vi "Stepper eSCL UDP.vi"(8 "error in":errorcluster, 9 "Axis Queue":refnum<queue>, 10 "UI Queue":refnum<queue>) -> (0 "error out":errorcluster)   [LabVIEW 2016, in "SMD-7615.lvlib"]
uses:
  SMD-7615.lvlib
  support/Message Queue/Message Cluster.ctl
  CTL/Stepper Drive Config.ctl
  CTL/SV General.ctl
  CTL/SV Inputs.ctl
  CTL/SV Outputs.ctl
  CTL/Motion IO.ctl
  CTL/Digital Lines (Read).ctl
  CTL/Status.ctl
  CTL/Encoder.ctl
  CTL/Position.ctl
  CTL/Axis Data.ctl
  support/Message Queue/Enqueue Message (Single).vi
  <vilib>/GPower/Error/Library/Append/AppendSingle.vi
  <vilib>/ErrorRing/Error Ring.xnode
  support/Message Queue/Message Queue.lvlib
  <vilib>/GPower/Error/GPError.lvlib
  LUL-All/LUL-Syslog/LUL-SysLog.lvlib
  eSCL/eSCL.lvlib
panel:
  out "DAQ time (ms)":u32
  out "Stall detected (Software)":bool
  out "Moving ? (Software)":bool
  out "Position":T1
  out "Encoder":T2
  out "Status":T3
  in  "Stop Button":bool
  out "Axis Name":string
  out "Digital Lines (Read)":T4
  out "Motion I/O":T5
  out "dt DAQ (ms)":u32
  out "Axis Config Constant":T6
  out "Last Received SV Update":timestamp
  out "Exit ?":bool
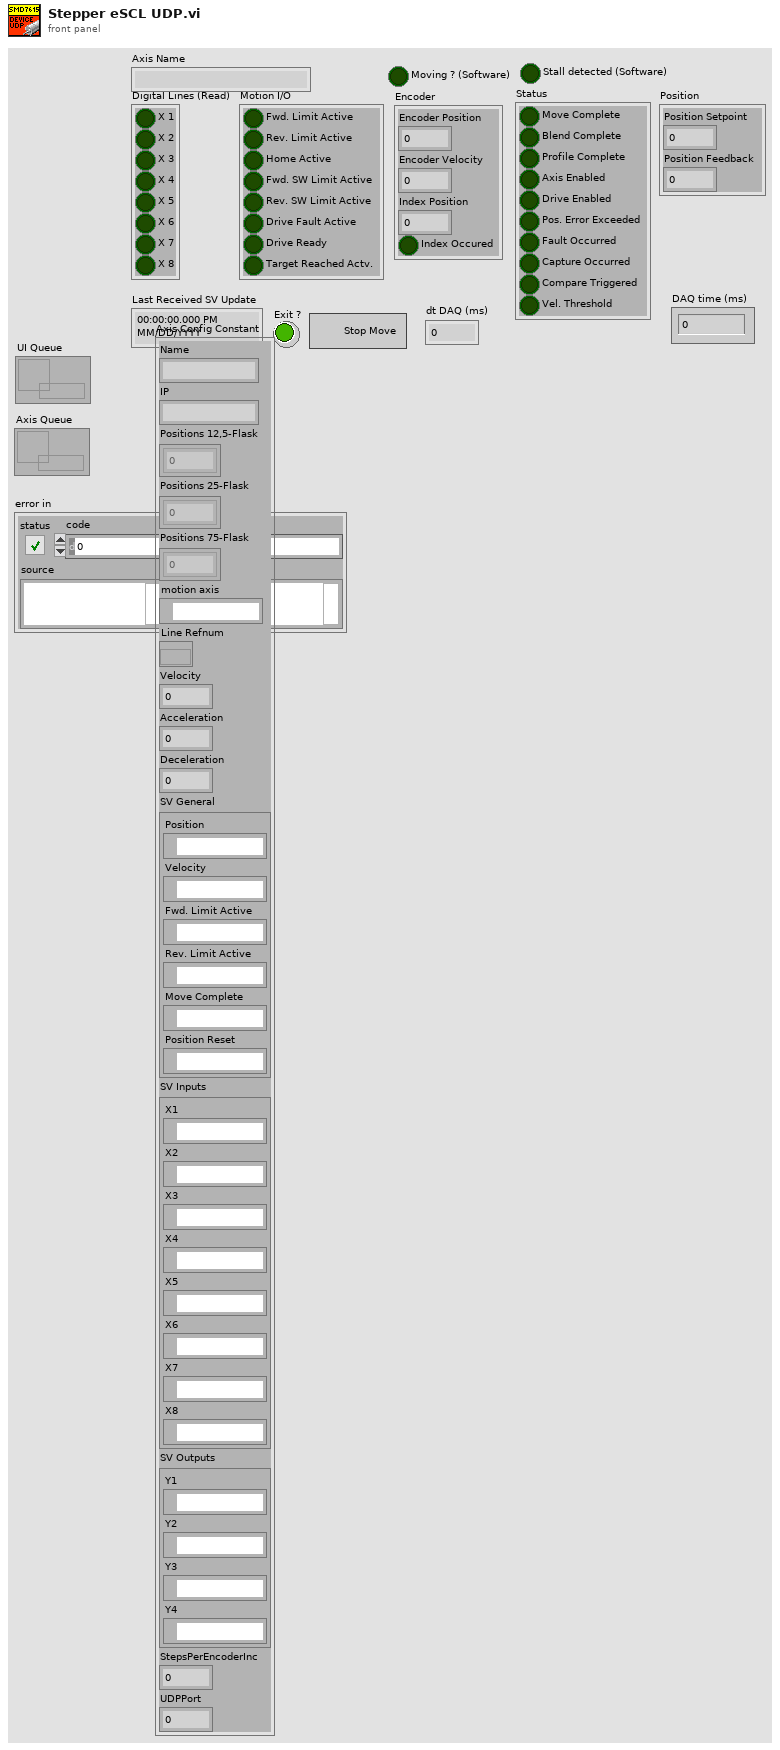
[diagram p1: front panel]
types:
  T1 = typedef "SMD-7615.lvlib/Position.ctl" = cluster{"Position Setpoint":dbl, "Position Feedback":dbl}
  T2 = typedef "SMD-7615.lvlib/Encoder.ctl" = cluster{"Encoder Position":dbl, "Encoder Velocity":dbl, "Index Position":dbl, "Index Occured":bool}
  T3 = typedef "SMD-7615.lvlib/Status.ctl" = cluster{"Move Complete":bool, "Blend Complete":bool, "Profile Complete":bool, "Axis Enabled":bool, "Drive Enabled":bool, "Pos. Error Exceeded":bool, "Fault Occurred":bool, "Capture Occurred":bool, "Compare Triggered":bool, "Vel. Threshold":bool}
  T4 = typedef "SMD-7615.lvlib/Digital Lines (Read).ctl" = cluster{"X 1":bool, "X 2":bool, "X 3":bool, "X 4":bool, "X 5":bool, "X 6":bool, "X 7":bool, "X 8":bool}
  T5 = typedef "SMD-7615.lvlib/Motion IO.ctl" = cluster{"Fwd. Limit Active":bool, "Rev. Limit Active":bool, "Home Active":bool, "Fwd. SW Limit Active":bool, "Rev. SW Limit Active":bool, "Drive Fault Active":bool, "Drive Ready":bool, "Target Reached Actv.":bool}
  T6 = typedef "SMD-7615.lvlib/Stepper Drive Config.ctl" = cluster{"Name":string, "IP":string, "Positions 12,5-Flask":dbl[], "Positions 25-Flask":dbl[], "Positions 75-Flask":dbl[], "motion axis ":refnum<k21>, "Line Refnum":refnum<k20>, "Velocity":dbl, "Acceleration":dbl, "Deceleration":dbl, "SV General":T7, "SV Inputs":T8, "SV Outputs":T9, "StepsPerEncoderInc":i32, "UDPPort":u16}
  T7 = typedef "SMD-7615.lvlib/SV General.ctl" = cluster{"Position":refnum<k21>, "Velocity":refnum<k21>, "Fwd. Limit Active":refnum<k21>, "Rev. Limit Active":refnum<k21>, "Move Complete":refnum<k21>, "Position Reset":refnum<k21>}
  T8 = typedef "SMD-7615.lvlib/SV Inputs.ctl" = cluster{"X1":refnum<k21>, "X2":refnum<k21>, "X3":refnum<k21>, "X4":refnum<k21>, "X5":refnum<k21>, "X6":refnum<k21>, "X7":refnum<k21>, "X8":refnum<k21>}
  T9 = typedef "SMD-7615.lvlib/SV Outputs.ctl" = cluster{"Y1":refnum<k21>, "Y2":refnum<k21>, "Y3":refnum<k21>, "Y4":refnum<k21>}
  T10 = typedef "SMD-7615.lvlib/Axis Data.ctl" = cluster{"Motion I/O":T5, "Digital Lines (Read)":T4, "Status":T3, "Encoder":T2, "Position":T1, "Moving ? (Software)":bool, "Stall detected (Software)":bool}
  T11 = typedef "LUL-SysLog.lvlib/SysLog Severity.ctl" = enum16{"Emergency", "Alert", "Critical", "Error", "Wanring", "Notice", "Informational", "Debug"}
  T12 = enum32{"Invalid", "Standard", "Closed", "Hidden", "Minimized", "Maximized"}
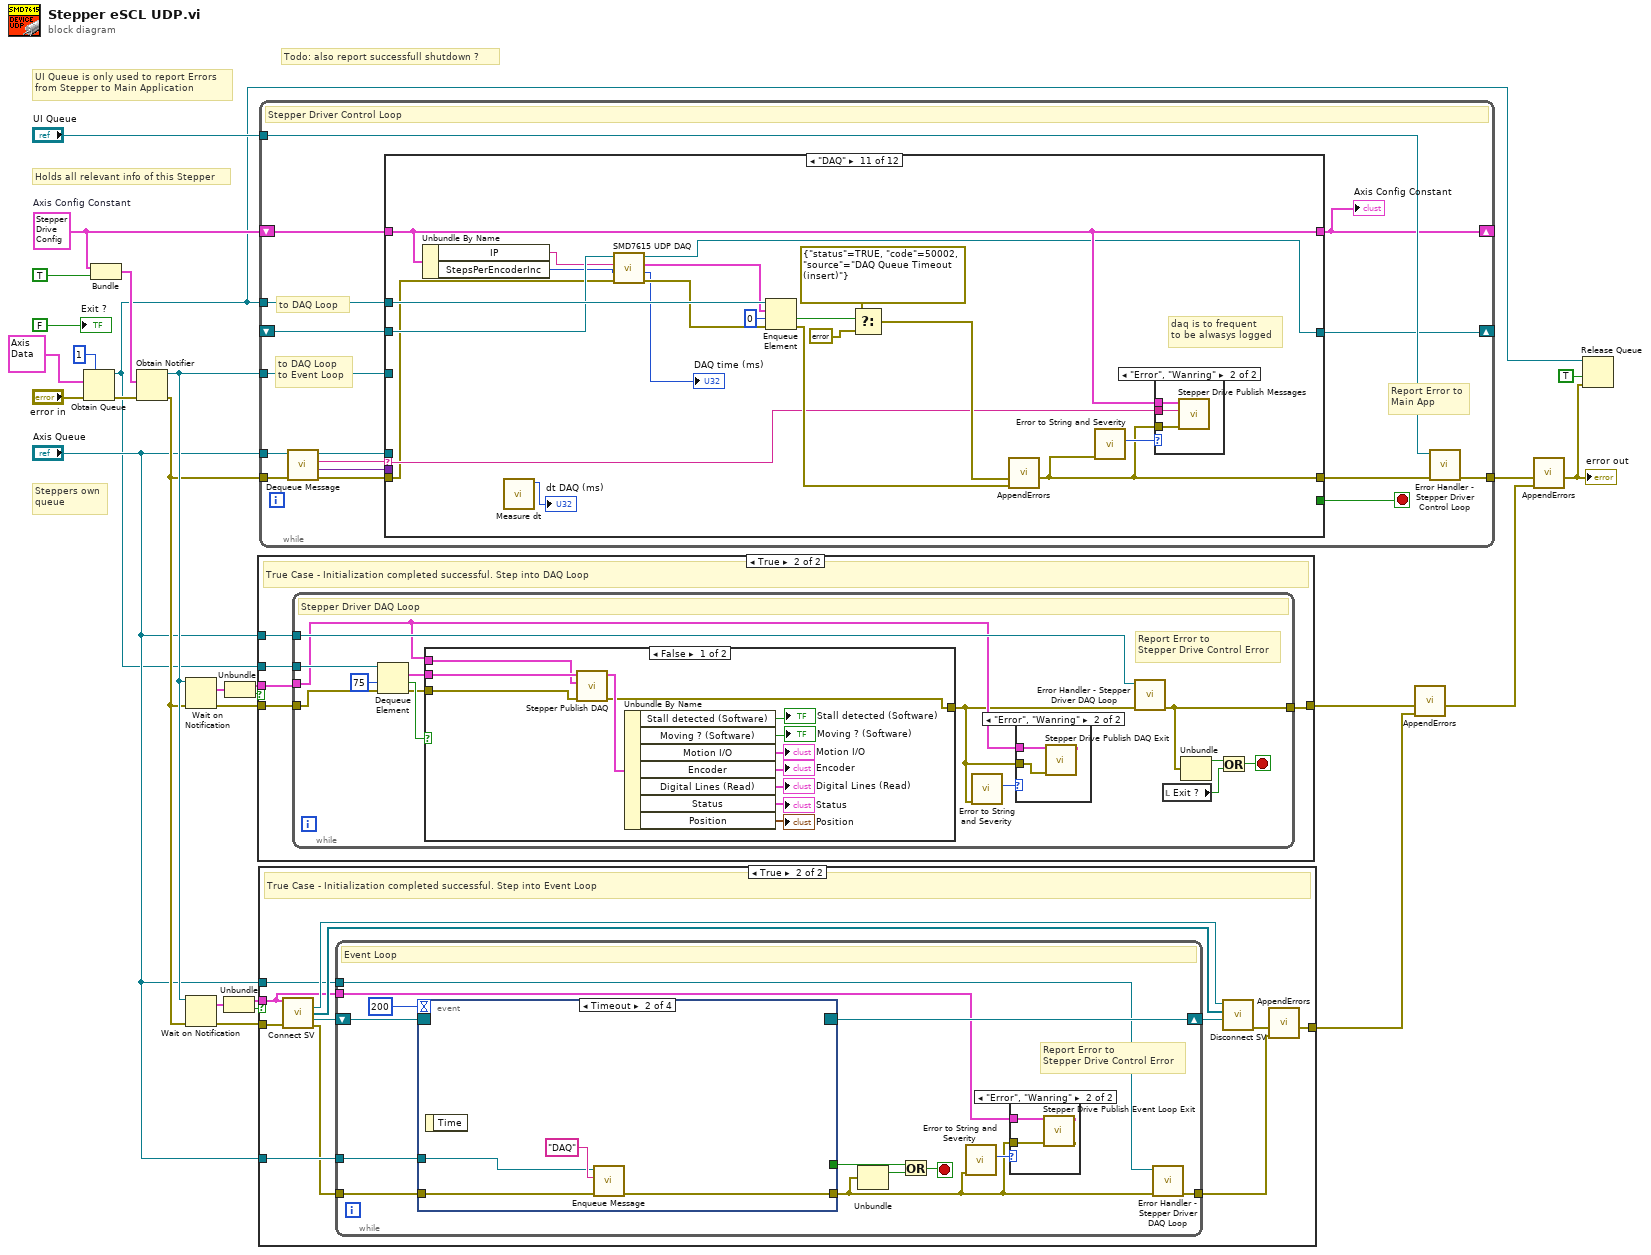
[diagram p0: block diagram]
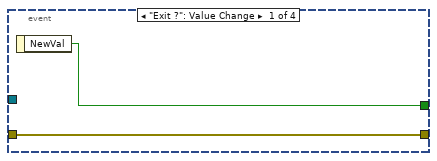
[diagram p4: hidden frame]
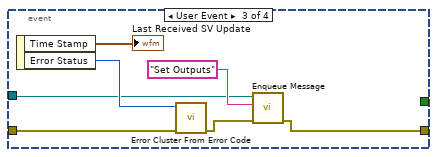
[diagram p5: hidden frame]
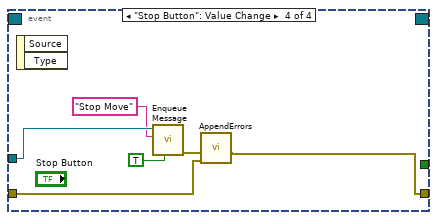
[diagram p6: hidden frame]
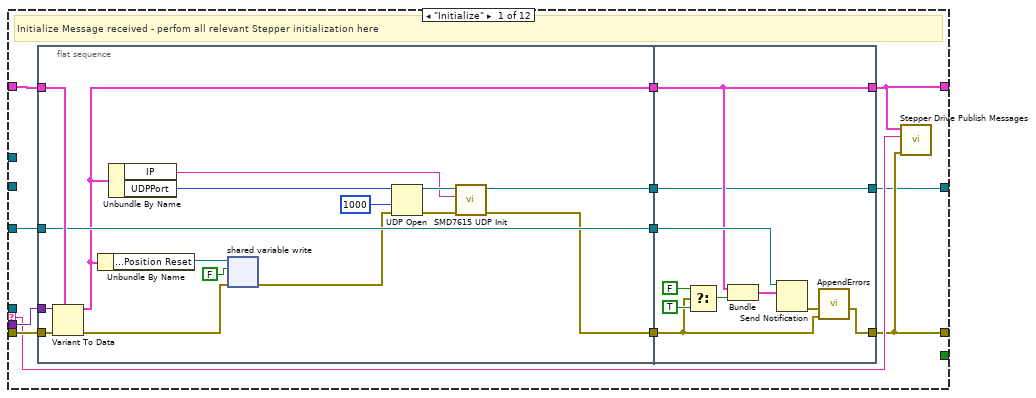
[diagram p10: hidden frame]
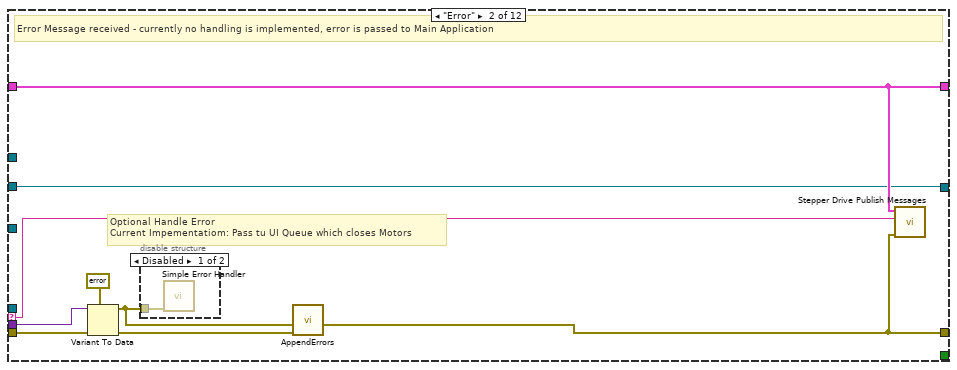
[diagram p11: hidden frame]
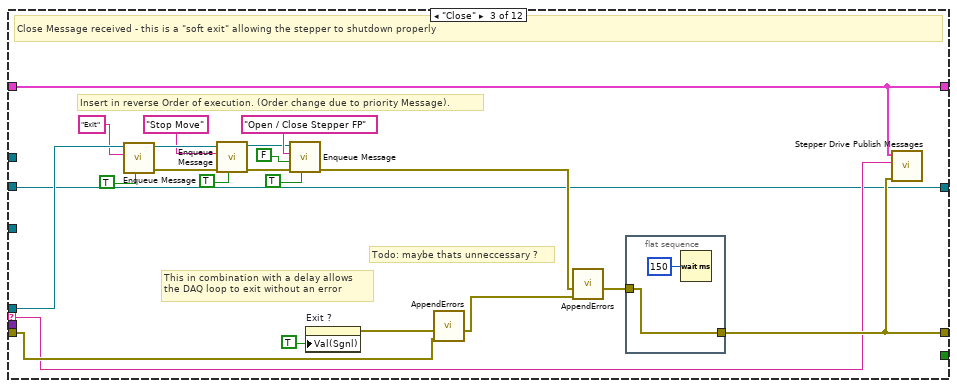
[diagram p13: hidden frame]
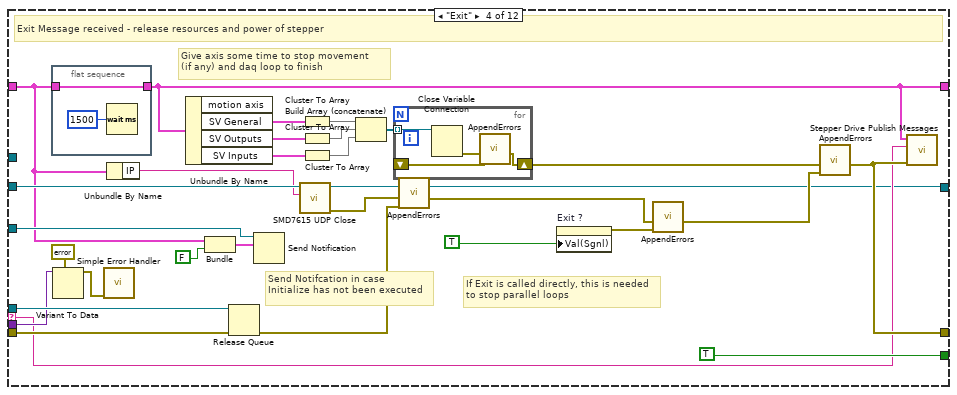
[diagram p14: hidden frame]
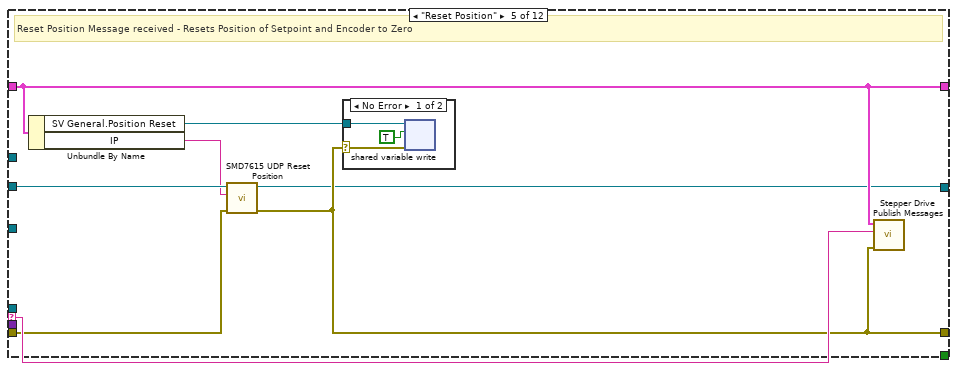
[diagram p15: hidden frame]
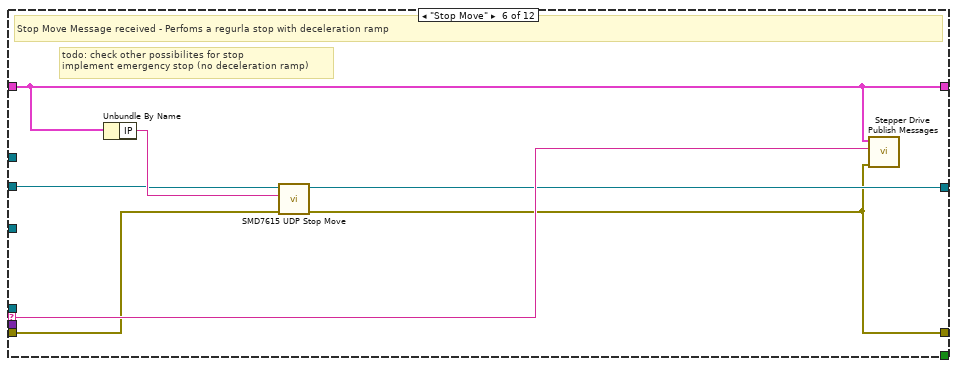
[diagram p17: hidden frame]
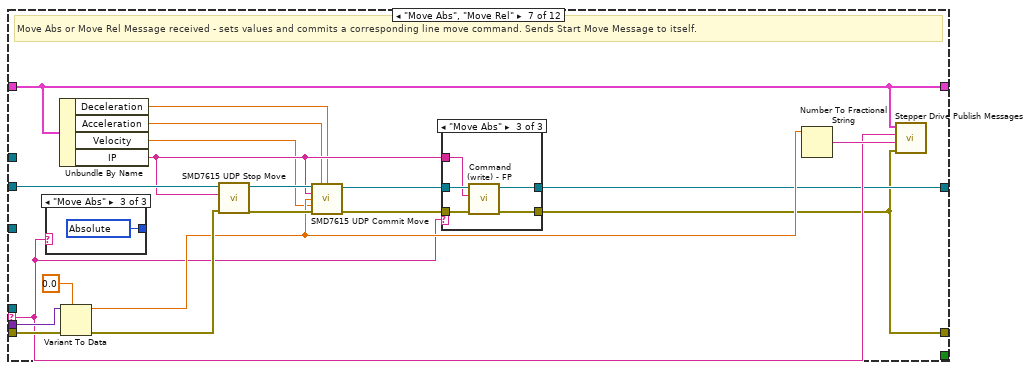
[diagram p18: hidden frame]
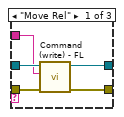
[diagram p19: hidden frame]
diagram:
  w12 = T6 {"Name"="", "IP"="", "Positions 12,5-Flask"=[], "Positions 25-Flask"=[], "Positions 75-Flask"=[], "motion axis "="", "Line Refnum"=refnum, "Velocity"=0.0, "Acceleration"=0.0, "Deceleration"=0.0, "SV General"={"Position"="", "Velocity"="", "Fwd. Limit Active"="", "Rev. Limit Active"="", "Move Complete"="", "Position Reset"=""}, "SV Inputs"={"X1"="", "X2"="", "X3"="", "X4"="", "X5"="", "X6"="", "X7"="", "X8"=""}, "SV Outputs"={"Y1"="", "Y2"="", "Y3"="", "Y4"=""}, "StepsPerEncoderInc"=0, "UDPPort"=0}  # Axis Config Constant
  # "Steppers own\nqueue"
  # "Holds all relevant info of this Stepper"
  # "Todo: also report successfull shutdown ?"
  # "UI Queue is only used to report Errors\nfrom Stepper to Main Application"
  n1 = Obtain Queue(max queue size (-1, unlimited)=1, element data type=T10 {"Motion I/O"={"Fwd. Limit Active"=FALSE, "Rev. Limit Active"=FALSE, "Home Active"=FALSE, "Fwd. SW Limit Active"=FALSE, "Rev. SW Limit Active"=FALSE, "Drive Fault Active"=FALSE, "Drive Ready"=FALSE, "Target Reached Actv."=FALSE}, "Digital Lines (Read)"={"X 1"=FALSE, "X 2"=FALSE, "X 3"=FALSE, "X 4"=FALSE, "X 5"=FALSE, "X 6"=FALSE, "X 7"=FALSE, "X 8"=FALSE}, "Status"={"Move Complete"=FALSE, "Blend Complete"=FALSE, "Profile Complete"=FALSE, "Axis Enabled"=FALSE, "Drive Enabled"=FALSE, "Pos. Error Exceeded"=FALSE, "Fault Occurred"=FALSE, "Capture Occurred"=FALSE, "Compare Triggered"=FALSE, "Vel. Threshold"=FALSE}, "Encoder"={"Encoder Position"=0.0, "Encoder Velocity"=0.0, "Index Position"=0.0, "Index Occured"=FALSE}, "Position"={"Position Setpoint"=0.0, "Position Feedback"=0.0}, "Moving ? (Software)"=FALSE, "Stall detected (Software)"=FALSE} ("Axis Data"), error in (no error)="error in") -> (queue out=w2:refnum<queue>, error out=w3:errorcluster)  [unwired: 2 in, 1 out]
  n2 = Bundle("Axis Config Constant"=w12, TRUE) -> (w23:cluster{"Axis Config Constant":T6, bool})  [unwired: 1 in]
  n3 = Obtain Notifier(notification data type=w23, error in (no error)=w3) -> (notifier out=w24:refnum<notifier>, error out=w11:errorcluster)  [unwired: 2 in, 1 out]
  n4 = Wait on Notification(notifier=w24, error in (no error)=w11) -> (notification=w21:cluster{"Axis Config Constant":T6, bool}, error out=w26:errorcluster)  [unwired: 2 in, 2 out]
  n5 = Wait on Notification(notifier=w24, error in (no error)=w11) -> (notification=w18:cluster{"Axis Config Constant":T6, bool}, error out=w25:errorcluster)  [unwired: 2 in, 2 out]
  n6 = Unbundle(w18) -> ("Axis Config Constant"=w16:T6, w17:bool)
  n7 = Unbundle(w21) -> ("Axis Config Constant"=w19:T6, w20:bool)
  n8 = case shown="True" w20 {
    tunnel: [w28 w33] -> w10
    tunnel: "Axis Queue" -> [_ w32]
    tunnel: w26 -> [w28 w31]
    tunnel: w19 -> [_ w30]
    tunnel: w2 -> [_ w29]
    frame False {
      # "False Case - Initialization not successful. Skip DAQ Loop"
    }
    frame True {
      # "True Case - Initialization completed successful. Step into DAQ Loop"
      n9 = while {
        tunnel: w31 -> [w40]
        tunnel: [w46] -> w33
        tunnel: w32 -> [w47]
        tunnel: w30 -> [w36]
        tunnel: w29 -> [w41]
        stop <- w43 stop-if-true
        # "Report Error to\nStepper Drive Control Error"
        # "Stepper Driver DAQ Loop"
        n10 = Dequeue Element(queue=w41, timeout in ms (-1)=75, error in (no error)=w40) -> (element=w42:T10, timed out?=w39:bool, error out=w37:errorcluster)  [unwired: 1 out]
        n11 = case shown="False" w39 {
          tunnel: [w51 w62] -> w35
          tunnel: w42 -> [w53 _]
          tunnel: w37 -> [w54 w62]
          tunnel: w36 -> [w50 _]
          frame False {
            n12 = call "Stepper Publish DAQ.vi"("error in"=w54, "BIBA 2017 Config"=w50, "Axis Data in"=w53) -> ("error out"=w51:errorcluster, "Axis Data out"=w52:T10)  [unwired: 7 in]
            n13 = Unbundle By Name(w52) -> ("Stall detected (Software)"=→"Stall detected (Software)":bool, "Moving ? (Software)"=→"Moving ? (Software)":bool, "Motion I/O"=→"Motion I/O":T5, "Encoder"=→"Encoder":T2, "Digital Lines (Read)"=→"Digital Lines (Read)":T4, "Status"=→"Status":T3, "Position"=→"Position":T1)
          }
          frame True {
          }
        }
        n14 = call "Error to String and Severity.vi"("error in (no error)"=w35) -> ("Severity"=w34:T11)  [unwired: 9 in, 1 out]
        n15 = case shown="\"Error\", \"Wanring\"" w34 {
          tunnel: w35 -> [_ w48]
          tunnel: w36 -> [_ w49]
          frame Default {
          }
          frame "Error", "Wanring" {
            n16 = call "Stepper Drive Publish DAQ Exit.vi"("error in (no error)"=w48, "Axis Config Constant"=w49) -> ()  [unwired: 10 in]
          }
        }
        n17 = call "Error Handler - Stepper Driver DAQ Loop.vi"("error in (no error)"=w35, "Message Queue"=w47) -> ("dup error in"=w46:errorcluster)  [unwired: 8 in, 1 out]
        n18 = local read "Exit ?"() -> (w44:bool)
        n19 = Unbundle(w46) -> ("status"=w45:bool)  [unwired: 2 out]
        n20 = Or(x=w45, y=w44) -> (x .or. y?=w43:bool)
      }
    }
  }
  n21 = case shown="True" w17 {
    tunnel: "Axis Queue" -> [_ w75]
    tunnel: [w63 w67] -> w9
    tunnel: w25 -> [w63 w74]
    tunnel: w16 -> [_ w64]
    tunnel: "Axis Queue" -> [_ w65]
    frame False {
      # "False Case - Initialization not successful. Skip Event Loop"
    }
    frame True {
      # "True Case - Initialization completed successful. Step into Event Loop"
      n22 = call "Connect SV.vi"("Axis Config in"=w64, "Error In"=w74) -> ("shared variable value change notification"=w71:refnum<user-event>, "Shared Variables"=w69:refnum<k21>[], "Event Registration Refnum"=w72:refnum<event-registration>, "Error Out"=w73:errorcluster)  [unwired: 9 in, 1 out]
      n23 = while {
        tunnel: w75 -> [w86]
        tunnel: w73 -> [w88]
        tunnel: [w81] -> w68
        shift-right: [w85] -> w70
        shift-left: w72 -> [w87]
        tunnel: w65 -> [w80]
        tunnel: w64 -> [w77]
        stop <- w83 stop-if-true
        # "Report Error to\nStepper Drive Control Error"
        # "Event Loop"
        n24 = event shown="[1] Timeout" {
          selector: w87 -> [_ _ _ _]
          dyn-events: [_ _ _ _] -> w85
          timeout: 200 ("Numeric") -> [_ _ _ _]
          tunnel: w88 -> [w92 w94 w101 w105]
          tunnel: [w92 w93 w97 w106] -> w76
          tunnel: w86 -> [_ w95 w99 w108]
          tunnel: [w91 _ _ _] -> w82
          event "Exit ?": Value Change {
            n25 = event-data() -> ("NewVal"=w91:bool)  [unwired: 1 in]
          }
          event Timeout {
            n26 = event-data() -> ()  [unwired: 1 in, 1 out]
            n27 = call-poly "Enqueue Message.vi"("error in (no error)"=w94, "Message"="DAQ", "Message Queue"=w95) -> ("error out"=w93:errorcluster)  [unwired: 7 in, 1 out]
          }
          event User Event {
            n28 = event-data() -> ("Time Stamp"=→"Last Received SV Update":timestamp, "Error Status"=w100:i32)  [unwired: 1 in]
            n29 = call <vilib>:"Error Cluster From Error Code.vi"("error in (no error)"=w101, "error code (0)"=w100) -> ("error out"=w102:errorcluster)  [unwired: 1 in, 6 out]
            n30 = call-poly "Enqueue Message.vi"("error in (no error)"=w102, "Message"="Set Outputs", "Message Queue"=w99) -> ("error out"=w97:errorcluster)  [unwired: 7 in, 1 out]
          }
          event "Stop Button": Value Change {
            n31 = event-data() -> ()  [unwired: 1 in, 2 out]
            n32 = call-poly "Enqueue Message.vi"("Priority Message? (F)"=TRUE, "Message"="Stop Move", "Message Queue"=w108) -> ("error out"=w104:errorcluster)  [unwired: 7 in, 1 out]
            n33 = call-poly <vilib>:"AppendErrors.vi"("Error to append"=w105, "Error in"=w104) -> ("Appended errors out"=w106:errorcluster)  [unwired: 9 in]
          }
        }
        n34 = Unbundle(w76) -> ("status"=w84:bool)  [unwired: 2 out]
        n35 = Or(x=w82, y=w84) -> (x .or. y?=w83:bool)
        n36 = call "Error to String and Severity.vi"("error in (no error)"=w76) -> ("Severity"=w78:T11)  [unwired: 9 in, 1 out]
        n37 = case shown="\"Error\", \"Wanring\"" w78 {
          tunnel: w76 -> [_ w89]
          tunnel: w77 -> [_ w90]
          frame Default {
          }
          frame "Error", "Wanring" {
            n38 = call "Stepper Drive Publish Event Loop Exit.vi"("error in (no error)"=w89, "Axis Config Constant"=w90) -> ()  [unwired: 10 in]
          }
        }
        n39 = call "Error Handler - Stepper Driver DAQ Loop.vi"("error in (no error)"=w76, "Message Queue"=w80) -> ("dup error in"=w81:errorcluster)  [unwired: 8 in, 1 out]
      }
      n40 = call "Disconnect SV.vi"("Event Registration Refnum"=w70, "Shared Variables"=w69, "User Event in"=w71) -> ("error out"=w66:errorcluster)  [unwired: 8 in]
      n41 = call-poly <vilib>:"AppendErrors.vi"("Error to append"=w68, "Error in"=w66) -> ("Appended errors out"=w67:errorcluster)  [unwired: 9 in]
    }
  }
  n42 = while {
    tunnel: "Axis Queue" -> [w125]
    tunnel: w11 -> [w124]
    tunnel: [w120] -> w14
    shift-right: [w116] -> _
    shift-left: w12 -> [w121]
    tunnel: "UI Queue" -> [w119]
    tunnel: w24 -> [w117]
    tunnel: w2 -> [w112]
    shift-right: [w111] -> _
    shift-left: _ -> [w110]
    stop <- w122 stop-if-true
    # "to DAQ Loop\nto Event Loop"
    # "to DAQ Loop"
    # "Report Error to\nMain App"
    # "Stepper Driver Control Loop"
    n43 = call "Dequeue Message.vi"("error in (no error)"=w124, "Message Queue"=w125) -> ("error out"=w114:errorcluster, "Message Data"=w123:variant, "Message"=w115:string, "dup Message Queue"=w118:refnum<queue>)  [unwired: 6 in]
    n44 = case shown="\"DAQ\"" w115 {
      selector: w115 -> [w129 w165 w175 w204 w240 w251 w260 w289 w291 w336 w364 w380]
      tunnel: w123 -> [w136 w171 _ w223 _ _ w268 _ _ w344 _ _]
      tunnel: w114 -> [w137 w170 w182 w225 w237 w247 w270 w287 w301 w345 w360 w381]
      tunnel: [w128 w167 w176 w206 w236 w248 w256 w287 w292 w337 w365 w379] -> w113
      tunnel: w118 -> [_ _ w195 w224 _ _ _ _ _ _ _ _]
      tunnel: [_ _ _ TRUE _ _ _ _ _ _ _ _] -> w122
      tunnel: w121 -> [w135 w166 w177 w201 w239 w250 w267 w288 w293 w338 w362 w378]
      tunnel: [w130 w166 w177 w205 w239 w250 w267 w288 w293 w338 w362 w378] -> w116
      tunnel: w117 -> [w131 _ _ w208 _ _ _ _ _ _ _ _]
      tunnel: w112 -> [_ _ _ _ _ _ _ _ _ _ w373 _]
      tunnel: [w127 w164 w174 w199 w234 w249 w257 w286 w290 w331 w358 w377] -> w111
      tunnel: w110 -> [_ w164 w174 w202 w238 w245 w265 w286 w290 w331 w363 w377]
      frame "Initialize" {
        # "Initialize Message received - perfom all relevant Stepper initialization here"
        n45 = flat-sequence {
          tunnel: w137 -> [w153]
          tunnel: w136 -> [w152]
          tunnel: w135 -> [w151]
          tunnel: [w139] -> w134
          tunnel: [w138] -> w133
          tunnel: [w150] -> w132
          tunnel: w131 -> [w150]
          tunnel: [w141] -> w126
          tunnel: [w155] -> w128
          tunnel: w134 -> [w156]
          tunnel: [w160] -> w130
          tunnel: w133 -> [w160]
          tunnel: w132 -> [w161]
          tunnel: [w154] -> w127
          tunnel: w126 -> [w154]
          frame #0 {
            n46 = Variant To Data(error in=w153, type=w151, Variant=w152) -> (data=w138:T6, error out=w147:errorcluster)
            n47 = Unbundle By Name(w138) -> ("SV General.Position Reset"=w148:refnum<k21>)
            n48 = Unbundle By Name(w138) -> ("IP"=w140:string, "UDPPort"=w144:u16)
            n49 = shared-variable-write(w148, w147, FALSE) -> (w146:errorcluster)  [unwired: 1 out]
            n50 = UDP Open(8:w146, 9:1000 ("timeout ms (25000)"), 11:w144) -> (port=w142:refnum<k16>, 0:w143:errorcluster)  [unwired: 2 in, 1 out]
            n51 = call "SMD7615 UDP Init.vi"("error in (no error)"=w143, "IP"=w140, "connection ID in"=w142) -> ("error out"=w139:errorcluster, "connection ID out"=w141:refnum<k16>)  [unwired: 7 in]
          }
          frame #1 {
            n52 = Select(t=FALSE ("Stepper Init Done"), s=w156, f=TRUE) -> (s? t:f=w159:bool)
            n53 = Bundle("Axis Config Constant"=w160, "f"=w159) -> (w158:cluster{"Axis Config Constant":T6, "f":bool})  [unwired: 1 in]
            n54 = Send Notification(notification=w158, notifier=w161) -> (error out=w157:errorcluster)  [unwired: 1 in, 1 out]
            n55 = call-poly <vilib>:"AppendErrors.vi"("Error to append"=w156, "Error in"=w157) -> ("Appended errors out"=w155:errorcluster)  [unwired: 9 in]
          }
        }
        n56 = call "Stepper Drive Publish Messages.vi"("error in (no error)"=w128, "Message"=w129, "Axis Config Constant"=w130) -> ()  [unwired: 9 in]
      }
      frame "Error" {
        # "Optional Handle Error\nCurrent Impementatiom: Pass tu UI Queue which closes Motors"
        # "Error Message received - currently no handling is implemented, error is passed to Main Application"
        n57 = Variant To Data(error in=w170, type=errorcluster {"status"=FALSE, "code"=0, "source"=""} ("error constant"), Variant=w171) -> (data=w169:errorcluster, error out=w168:errorcluster)
        n58 = disable-structure shown="Disabled" {
          disable-tunnel: w169 -> [w173 _]
          frame Disabled {
            n59 = call <vilib>:"Simple Error Handler.vi"("error in (no error)"=w173) -> ()  [unwired: 4 in, 5 out]
          }
          frame Enabled {
          }
        }
        n60 = call-poly <vilib>:"AppendErrors.vi"("Error to append"=w168, "Error in"=w169) -> ("Appended errors out"=w167:errorcluster)  [unwired: 9 in]
        n61 = call "Stepper Drive Publish Messages.vi"("error in (no error)"=w167, "Message"=w165, "Axis Config Constant"=w166) -> ()  [unwired: 9 in]
      }
      frame "Close" {
        # "Todo: maybe thats unneccessary ?"
        # "This in combination with a delay allows\nthe DAQ loop to exit without an error"
        # "Insert in reverse Order of execution. (Order change due to priority Message)."
        # "Close Message received - this is a \"soft exit\" allowing the stepper to shutdown properly"
        n62 = call-poly "Enqueue Message.vi"("Priority Message? (F)"=TRUE, "Message"="Exit", "Message Queue"=w195) -> ("error out"=w190:errorcluster, "dup Message Queue"=w191:refnum<queue>)  [unwired: 7 in]
        n63 = call-poly "Enqueue Message.vi"("Priority Message? (F)"=TRUE, "error in (no error)"=w190, "Message"="Stop Move", "Message Queue"=w191) -> ("error out"=w185:errorcluster, "dup Message Queue"=w186:refnum<queue>)  [unwired: 6 in]
        n64 = call-poly "Enqueue Message.vi"("Priority Message? (F)"=TRUE, "error in (no error)"=w185, "Message Data"=FALSE, "Message"="Open / Close Stepper FP", "Message Queue"=w186) -> ("error out"=w180:errorcluster)  [unwired: 5 in, 1 out]
        n65 = property on="Exit ?" class="Bool (strict)"("Val(Sgnl)"=TRUE ("Value (Signaling)")) -> (error out=w183:errorcluster)  [unwired: 2 in, 1 out]
        n66 = call-poly <vilib>:"AppendErrors.vi"("Error to append"=w182, "Error in"=w183) -> ("Appended errors out"=w179:errorcluster)  [unwired: 9 in]
        n67 = call-poly <vilib>:"AppendErrors.vi"("Error to append"=w179, "Error in"=w180) -> ("Appended errors out"=w181:errorcluster)  [unwired: 9 in]
        n68 = flat-sequence {
          tunnel: [w196] -> w176
          tunnel: w181 -> [w196]
          frame #0 {
            n69 = Wait (ms)(milliseconds to wait=u32 150) -> ()  [unwired: 1 out]
          }
        }
        n70 = call "Stepper Drive Publish Messages.vi"("error in (no error)"=w176, "Message"=w175, "Axis Config Constant"=w177) -> ()  [unwired: 9 in]
      }
      frame "Exit" {
        # "Send Notifcation in case\nInitialize has not been executed"
        # "Give axis some time to stop movement \n(if any) and daq loop to finish"
        # "If Exit is called directly, this is needed\nto stop parallel loops"
        # "Exit Message received - release resources and power of stepper"
        n71 = flat-sequence {
          tunnel: w201 -> [w228]
          tunnel: [w228] -> w205
          frame #0 {
            n72 = Wait (ms)(milliseconds to wait=u32 1500) -> ()  [unwired: 1 out]
          }
        }
        n73 = Variant To Data(type=errorcluster {"status"=FALSE, "code"=0, "source"=""} ("error constant"), Variant=w223) -> (data=w226:errorcluster)  [unwired: 1 in, 1 out]
        n74 = call <vilib>:"Simple Error Handler.vi"("error in (no error)"=w226) -> ()  [unwired: 4 in, 5 out]
        n75 = Unbundle By Name(w201) -> ("IP"=w200:string)
        n76 = Unbundle By Name(w205) -> ("SV General"=w222:T7, "SV Outputs"=w218:T9, "SV Inputs"=w219:T8)  [unwired: 1 out]
        n77 = Bundle("Axis Config Constant"=w201, FALSE) -> (w209:cluster{"Axis Config Constant":T6, bool})  [unwired: 1 in]
        n78 = Release Queue(queue=w224, error in (no error)=w225) -> (error out=w213:errorcluster)  [unwired: 1 in, 2 out]
        n79 = Send Notification(notification=w209, notifier=w208) -> ()  [unwired: 1 in, 2 out]
        n80 = call "SMD7615 UDP Close.vi"("IP"=w200, "connection ID in"=w202) -> ("error out"=w203:errorcluster, "connection ID out"=w199:refnum<k16>)  [unwired: 8 in]
        n81 = Cluster To Array(cluster=w222) -> (array=w221:refnum<k21>[])
        n82 = Cluster To Array(cluster=w218) -> (array=w217:refnum<k21>[])
        n83 = Cluster To Array(cluster=w219) -> (array=w216:refnum<k21>[])
        n84 = Build Array (concatenate)(w221, w217, w216) -> (w220:refnum<k21>[])
        n85 = for {
          tunnel: w220 -> [w233] mode=indexing
          shift-right: [w231] -> w198
          shift-left: _ -> [w230]
          n86 = Close Variable Connection(11:w233) -> (0:w232:errorcluster)  [unwired: 1 in]
          n87 = call-poly <vilib>:"AppendErrors.vi"("Error to append"=w230, "Error in"=w232) -> ("Appended errors out"=w231:errorcluster)  [unwired: 9 in]
        }
        n88 = call-poly <vilib>:"AppendErrors.vi"("Error to append"=w213, "Error in"=w203) -> ("Appended errors out"=w211:errorcluster)  [unwired: 9 in]
        n89 = property on="Exit ?" class="Bool (strict)"("Val(Sgnl)"=TRUE ("Value (Signaling)")) -> (error out=w212:errorcluster)  [unwired: 2 in, 1 out]
        n90 = call-poly <vilib>:"AppendErrors.vi"("Error to append"=w212, "Error in"=w211) -> ("Appended errors out"=w210:errorcluster)  [unwired: 9 in]
        n91 = call-poly <vilib>:"AppendErrors.vi"("Error to append"=w210, "Error in"=w198) -> ("Appended errors out"=w206:errorcluster)  [unwired: 9 in]
        n92 = call "Stepper Drive Publish Messages.vi"("error in (no error)"=w206, "Message"=w204, "Axis Config Constant"=w205) -> ()  [unwired: 9 in]
      }
      frame "Reset Position" {
        # "Reset Position Message received - Resets Position of Setpoint and Encoder to Zero"
        n93 = Unbundle By Name(w239) -> ("SV General.Position Reset"=w241:refnum<k21>, "IP"=w235:string)
        n94 = call "SMD7615 UDP Reset Position.vi"("error in (no error)"=w237, "IP"=w235, "connection ID in"=w238) -> ("error out"=w236:errorcluster, "connection ID out"=w234:refnum<k16>)  [unwired: 7 in]
        n95 = case shown="No Error" w236 {
          selector: w236 -> [w243 _]
          tunnel: w241 -> [w244 _]
          frame No Error {
            n96 = shared-variable-write(w244, w243, TRUE) -> ()  [unwired: 2 out]
          }
          frame Error {
          }
        }
        n97 = call "Stepper Drive Publish Messages.vi"("error in (no error)"=w236, "Message"=w240, "Axis Config Constant"=w239) -> ()  [unwired: 9 in]
      }
      frame "Stop Move" {
        # "todo: check other possibilites for stop\nimplement emergency stop (no deceleration ramp)"
        # "Stop Move Message received - Perfoms a regurla stop with deceleration ramp"
        n98 = Unbundle By Name(w250) -> ("IP"=w246:string)
        n99 = call "SMD7615 UDP Stop Move.vi"("error in (no error)"=w247, "IP"=w246, "connection ID in"=w245) -> ("error out"=w248:errorcluster, "connection ID out"=w249:refnum<k16>)  [unwired: 7 in]
        n100 = call "Stepper Drive Publish Messages.vi"("error in (no error)"=w248, "Message"=w251, "Axis Config Constant"=w250) -> ()  [unwired: 9 in]
      }
      frame "Move Abs", "Move Rel" {
        # "Move Abs or Move Rel Message received - sets values and commits a corresponding line move command. Sends Start Move Message to itself."
        n101 = case shown="\"Move Abs\"" w260 {
          tunnel: [w283 -1 ("Move Mode") w285] -> _
          frame "Move Rel" {
            w283 = 10551344 items=["Absolute"=10551337, "Relative"=10551344, "Relative To Capture"=10551345, "Velocity"=10551346] ("Move Mode")
          }
          frame Default {
          }
          frame "Move Abs" {
            w285 = 10551337 items=["Absolute"=10551337, "Relative"=10551344, "Relative To Capture"=10551345, "Velocity"=10551346] ("Move Mode")
          }
        }
        n102 = Unbundle By Name(w267) -> ("Deceleration"=w252:dbl, "Acceleration"=w253:dbl, "Velocity"=w254:dbl, "IP"=w255:string)
        n103 = Variant To Data(error in=w270, type=0.0 ("Position"), Variant=w268) -> (data=w261:dbl, error out=w264:errorcluster)
        n104 = call "SMD7615 UDP Stop Move.vi"("error in (no error)"=w264, "IP"=w255, "connection ID in"=w265) -> ("error out"=w262:errorcluster, "connection ID out"=w263:refnum<k16>)  [unwired: 7 in]
        n105 = call "SMD7615 UDP Commit Move.vi"("connection ID in"=w263, "Acceleration"=w253, "Deceleration"=w252, "IP"=w255, "Distance / Position"=w261, "Velocity"=w254, "error in (no error)"=w262) -> ("connection ID out"=w258:refnum<k16>, "error out"=w259:errorcluster)  [unwired: 7 in]
        n106 = case shown="\"Move Abs\"" w260 {
          tunnel: w259 -> [w274 w276 w282]
          tunnel: w258 -> [w275 w277 w281]
          tunnel: [w273 w277 w280] -> w257
          tunnel: [w272 w276 w279] -> w256
          tunnel: w255 -> [w271 _ w278]
          frame "Move Rel" {
            n107 = call "Command (write) - FL.vi"("error in (no error)"=w274, "IP"=w271, "connection ID in"=w275) -> ("error out"=w272:errorcluster, "connection ID out"=w273:refnum<k16>)  [unwired: 7 in]
          }
          frame Default {
          }
          frame "Move Abs" {
            n108 = call "Command (write) - FP.vi"("error in (no error)"=w282, "IP"=w278, "connection ID in"=w281) -> ("error out"=w279:errorcluster, "connection ID out"=w280:refnum<k16>)  [unwired: 7 in]
          }
        }
        n109 = Number To Fractional String(number=w261) -> (F-format string=w266:string)  [unwired: 3 in]
        n110 = call "Stepper Drive Publish Messages.vi"("error in (no error)"=w256, "Parameter"=w266, "Message"=w260, "Axis Config Constant"=w267) -> ()  [unwired: 8 in]
      }
      frame "Start Move" {
        # "not present in udp version"
        # "Start move Message received - Start the previously commited line move"
        n111 = call "Stepper Drive Publish Messages.vi"("error in (no error)"=w287, "Message"=w289, "Axis Config Constant"=w288) -> ()  [unwired: 9 in]
      }
      frame "Set Outputs" {
        w313 = TRUE
        # "Set Outputs Message received - Output values come from shared variables. If any changes all are set."
        n112 = Unbundle By Name(w293) -> ("IP"=w303:string, "SV Outputs.Y1"=w312:refnum<k21>, "SV Outputs.Y2"=w311:refnum<k21>, "SV Outputs.Y3"=w310:refnum<k21>, "SV Outputs.Y4"=w309:refnum<k21>)
        n113 = shared-variable-read(w312, w313) -> (w300:errorcluster, w308:bool)  [unwired: 1 in, 2 out]
        n114 = shared-variable-read(w311, w313) -> (w299:errorcluster, w307:bool)  [unwired: 1 in, 2 out]
        n115 = shared-variable-read(w310, w313) -> (w298:errorcluster, w306:bool)  [unwired: 1 in, 2 out]
        n116 = shared-variable-read(w309, w313) -> (w297:errorcluster, w305:bool)  [unwired: 1 in, 2 out]
        n117 = call-poly <vilib>:"AppendErrors.vi"("Error to append"=w299, "Error in"=w300) -> ("Appended errors out"=w296:errorcluster)  [unwired: 9 in]
        n118 = call-poly <vilib>:"AppendErrors.vi"("Error to append"=w297, "Error in"=w298) -> ("Appended errors out"=w294:errorcluster)  [unwired: 9 in]
        n119 = Build Array(w308, w307, w306, w305) -> (w304:bool[])
        n120 = call-poly <vilib>:"AppendErrors.vi"("Error to append"=w294, "Error in"=w296) -> ("Appended errors out"=w295:errorcluster)  [unwired: 9 in]
        n121 = for {
          tunnel: w304 -> [w319] mode=indexing
          tunnel: w303 -> [w314]
          shift-right: [w315] -> w302
          shift-left: w295 -> [w317]
          tunnel: w290 -> [w318]
          i -> [w320]
          n122 = Increment(x=w320) -> (x+1=w316:i32)
          n123 = case shown="True" w319 {
            tunnel: w318 -> [w324 w330]
            tunnel: w317 -> [w323 w329]
            tunnel: w316 -> [w322 w328]
            tunnel: [w325 w327] -> w315
            tunnel: w314 -> [w321 w326]
            frame False {
              n124 = call "Command (write) - IL.vi"("error in (no error)"=w323, "Output"=w322, "IP"=w321, "connection ID in"=w324) -> ("error out"=w325:errorcluster)  [unwired: 6 in, 1 out]
            }
            frame True {
              n125 = call "Command (write) - IH.vi"("error in (no error)"=w329, "Output"=w328, "IP"=w326, "connection ID in"=w330) -> ("error out"=w327:errorcluster)  [unwired: 6 in, 1 out]
            }
          }
        }
        n126 = call-poly <vilib>:"AppendErrors.vi"("Error to append"=w301, "Error in"=w302) -> ("Appended errors out"=w292:errorcluster)  [unwired: 9 in]
        n127 = call "Stepper Drive Publish Messages.vi"("error in (no error)"=w292, "Message"=w291, "Axis Config Constant"=w293) -> ()  [unwired: 9 in]
      }
      frame "Open / Close Stepper FP" {
        # "Open / Close Stepper FP Message received - Opens or closes VI Frontpanel. This is intended to be a debugging feature"
        n128 = Unbundle By Name(w338) -> ("Name"=→"Axis Name":string)
        n129 = control-ref of="This VI"() -> (w342:refnum<vi>)
        n130 = Variant To Data(error in=w345, type=TRUE, Variant=w344) -> (data=w333:bool, error out=w339:errorcluster)
        n131 = case shown="False" w333 {
          tunnel: w342 -> [w349 w351]
          tunnel: [w348 w350] -> w340
          frame False {
            # "1149: cannot close \nclosed frontpanel"
            n132 = invoke class="VI" method="FP.Close"(reference=w349) -> (error out=w347:errorcluster)  [unwired: 2 in, 2 out]
            n133 = call <vilib>:"Clear Errors.vi"("error in (no error)"=w347, "specific error code to clear (0: all)"=1149) -> ("error out"=w348:errorcluster)  [unwired: 4 in, 1 out]
          }
          frame True {
            n134 = invoke class="VI" method="FP.Open"(reference=w351, "Activate"=TRUE ("Activate?"), "State"=T12."Standard") -> (error out=w350:errorcluster)  [unwired: 2 in, 4 out]
          }
        }
        n135 = call-poly <vilib>:"AppendErrors.vi"("Error to append"=w339, "Error in"=w340) -> ("Appended errors out"=w337:errorcluster)  [unwired: 9 in]
        n136 = Select(t="True", s=w333, f="False") -> (s? t:f=w332:string)
        n137 = call "Stepper Drive Publish Messages.vi"("error in (no error)"=w337, "Parameter"=w332, "Message"=w336, "Axis Config Constant"=w338) -> ()  [unwired: 8 in]
      }
      frame "DAQ" {
        # "daq is to frequent\nto be alwasys logged"
        n138 = Unbundle By Name(w362) -> ("IP"=w361:string, "StepsPerEncoderInc"=w354:i32)
        n139 = call "Measure dt.vi"() -> ("dt"=→"dt DAQ (ms)":u32)  [unwired: 11 in]
        n140 = call "SMD7615 UDP DAQ.vi"("error in (no error)"=w360, "StepsPerEncoderInc"=w354, "IP"=w361, "connection ID in"=w363) -> ("error out"=w359:errorcluster, "DAQ time (ms)"=→"DAQ time (ms)":u32, "DAQ Data"=w355:T10, "connection ID out"=w358:refnum<k16>)  [unwired: 4 in]
        n141 = Enqueue Element(queue=w373, element=w355, timeout in ms (-1)=0, error in (no error)=w359) -> (timed out?=w371:bool, error out=w367:errorcluster)  [unwired: 1 out]
        n142 = Select(t=errorcluster {"status"=TRUE, "code"=50002, "source"="DAQ Queue Timeout (insert)"}, s=w371, f=errorcluster {"status"=FALSE, "code"=0, "source"=""} ("error in (no error)")) -> (s? t:f=w370:errorcluster)
        n143 = call-poly <vilib>:"AppendErrors.vi"("Error to append"=w367, "Error in"=w370) -> ("Appended errors out"=w365:errorcluster)  [unwired: 9 in]
        n144 = call "Error to String and Severity.vi"("error in (no error)"=w365) -> ("Severity"=w366:T11)  [unwired: 9 in, 1 out]
        n145 = case shown="\"Error\", \"Wanring\"" w366 {
          tunnel: w365 -> [_ w376]
          tunnel: w362 -> [_ w375]
          tunnel: w364 -> [_ w374]
          frame Default {
          }
          frame "Error", "Wanring" {
            n146 = call "Stepper Drive Publish Messages.vi"("error in (no error)"=w376, "Message"=w374, "Axis Config Constant"=w375) -> ()  [unwired: 9 in]
          }
        }
      }
      frame Default {
        # "Anything else received - This is invalid and handled as an Error"
        n147 = Unbundle By Name(w378) -> ("Name"=w383:string)
        n148 = xnode "Error Ring"("parameter 0"=w380, "parameter 1"=w383) -> ("error out"=w382:errorcluster)
        n149 = call-poly <vilib>:"AppendErrors.vi"("Error to append"=w381, "Error in"=w382) -> ("Appended errors out"=w379:errorcluster)  [unwired: 9 in]
        n150 = call "Stepper Drive Publish Messages.vi"("error in (no error)"=w379, "Message"=w380, "Axis Config Constant"=w378) -> ()  [unwired: 9 in]
      }
    }
    "Axis Config Constant" <- w116
    n151 = call "Error Handler - Stepper Driver Control Loop.vi"("error in (no error)"=w113, "Message Queue"=w119) -> ("dup error in"=w120:errorcluster)  [unwired: 8 in, 1 out]
  }
  n152 = call-poly <vilib>:"AppendErrors.vi"("Error to append"=w9, "Error in"=w10) -> ("Appended errors out"=w13:errorcluster)  [unwired: 9 in]
  n153 = call-poly <vilib>:"AppendErrors.vi"("Error to append"=w13, "Error in"=w14) -> ("Appended errors out"=w4:errorcluster)  [unwired: 9 in]
  "error out" <- w4
  n154 = Release Queue(queue=w2, force destroy? (F)=TRUE, error in (no error)=w4) -> ()  [unwired: 3 out]
  "Exit ?" <- FALSE ("Exit ?")
